vi "Distance-Velocity from Freq.vi"(0 "freq_rising":dbl, 2 "Empirical Distance Costant":dbl=4.28571429e-07 format="%#_13g", 3 "freq_falling":dbl) -> (5 "Distance (m)":dbl, 6 "Mean Frequency":dbl, 7 "Velocity (m/s)":dbl)   [LabVIEW 2014]
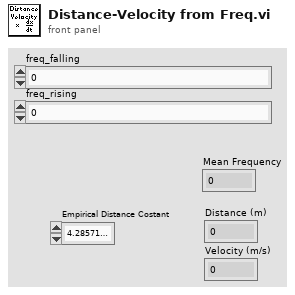
[diagram p1: front panel]
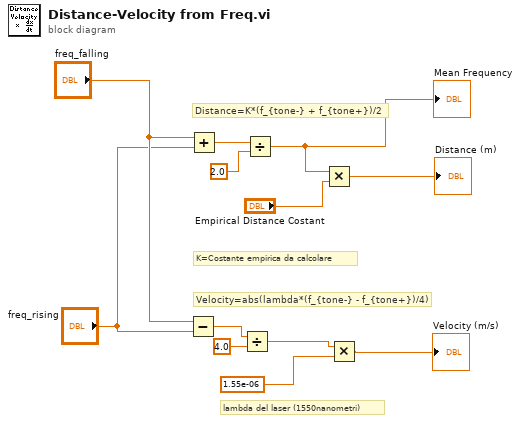
[diagram p0: block diagram]
diagram:
  # "Velocity=abs(lambda*(f_{tone-} - f_{tone+})/4)"
  # "Distance=K*(f_{tone-} + f_{tone+})/2"
  # "lambda del laser (1550nanometri)"
  # "K=Costante empirica da calcolare"
  n1 = Subtract(x="freq_falling", y="freq_rising") -> (x-y=w7:dbl)
  n2 = Add(x="freq_falling", y="freq_rising") -> (x+y=w12:dbl)
  n3 = Divide(x=w7, y=4.0) -> (x/y=w5:dbl)
  n4 = Divide(x=w12, y=2.0) -> (x/y=w10:dbl)
  "Mean Frequency" <- w10
  n5 = Multiply(x=w10, y="Empirical Distance Costant") -> (x*y=→"Distance (m)":dbl)
  n6 = Multiply(x=w5, y=1.55e-06) -> (x*y=→"Velocity (m/s)":dbl)
